vi "W1Q1.vi"() -> ()   [LabVIEW 2021]
panel:
  out "Numeric 2":dbl
  in  "Numeric":dbl
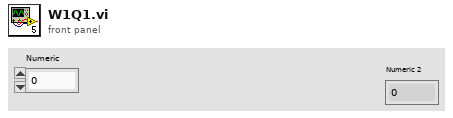
[diagram p1: front panel]
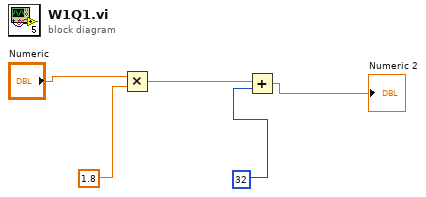
[diagram p0: block diagram]
diagram:
  n1 = Multiply(x="Numeric", y=1.8) -> (x*y=w3:dbl)
  n2 = Add(x=w3, y=32) -> (x+y=→"Numeric 2":dbl)
